vi "trialsExp.vi"() -> ()   [LabVIEW 2010]
uses:
  <instrlib>/niHWS/nihws.llb/niHWS Open File Permissions ID.ctl
  Statechart 1.lvsc/Trigger.ctl
  Statechart 1.lvsc/Inputs.ctl
  <vilib>/sound2/lvsound2.llb/Sound Data Format.ctl
  <vilib>/sound2/lvsound2.llb/Sampling Mode.ctl
  <vilib>/Statechart/Infrastructure/RTStatechart/RunTime SCN.xnode
  Statechart 1.lvsc/Outputs.ctl
  Statechart 1.lvsc
  <vilib>/Statechart/Common/IntGuid.ctl
  <vilib>/Statechart/Common/DbgID.ctl
  <vilib>/DAQmx/write.llb/DAQmx Write (Digital Bool 1Line 1Point).vi
  <instrlib>/niHWS/nihws.llb/niHWS Write Analog DBL.vi
  <vilib>/imath/engines/lvmath2/RunTimeEngine/ErrorHandling/NIMS_Finalize Error.vi
  <vilib>/imath/engines/lvmath2/RunTimeEngine/NodeEndStatement/NIMS_NodeEndStatement_Get Vector.vi
  <instcachedir>/0/NIMS_NodeEndStatement_Get Vector_F420F1081A35401FA339BC91980782B0.lvgen/NIMS_NodeEndStatement_Get Vector_F420F1081A35401FA339BC91980782B0_002.vi
  <vilib>/imath/engines/lvmath/Functions/Error Handling/MergeErrorsWrapper.vi
  <vilib>/imath/engines/lvmath2/RunTimeEngine/NodeEndStatement/NIMS_NodeEndStatement_Output.vi
  <instcachedir>/0/NIMS_NodeEndStatement_Output_53EC0D466D134D7ABD903AC30B43404B.lvgen/NIMS_NodeEndStatement_Output_53EC0D466D134D7ABD903AC30B43404B_004.vi
  <instcachedir>/0/NIMS_NodeEndStatement_Output_53EC0D466D134D7ABD903AC30B43404B.lvgen/NIMS_NodeEndStatement_Output_53EC0D466D134D7ABD903AC30B43404B_005.vi
  <vilib>/imath/engines/lvmath2/RunTimeEngine/RangeToken/NIMS_Range.vi
  <instcachedir>/0/NIMS_Range_1C63927E4E474DADACDA97C3F2261A11.lvgen/NIMS_Range_1C63927E4E474DADACDA97C3F2261A11_000.vi
  <vilib>/imathl/engines/lvmath/Functions/Error Handling/Create Error.vi
  <vilib>/imath/engines/lvmath2/RunTimeEngine/BuiltInFunctions/repeatmx/NIMS_repeatmx(GM, I32, I32).vi
  <instcachedir>/0/NIMS_repeatmx(GM, I32, I32)_69DEE8FEFC4F4D9AB51BA55E85245ECE.lvgen/NIMS_repeatmx(GM, I32, I32)_69DEE8FEFC4F4D9AB51BA55E85245ECE_004.vi
  <vilib>/imath/engines/lvmath2/RunTimeEngine/BuiltInFunctions/randpermutation/NIMS_randpermutation.vi
  <vilib>/imath/engines/lvmath2/RunTimeEngine/VariableToken/Read/NIMS_Get Elements - SorM(_) - Check.vi
  <instcachedir>/0/NIMS_Get Elements - SorM(_) - Check_404BE36992094B78AAADB7BD5278D7E3.lvgen/NIMS_Get Elements - SorM(_) - Check_404BE36992094B78AAADB7BD5278D7E3_006.vi
  <vilib>/sound2/lvsound2.llb/Sound Output Write (DBL Single).vi
  Statechart 1.lvsc/CompanionDiagram.vi/21/SC Main.vi
  <vilib>/daqmx/miscellaneous.llb/DAQmx Fill In Error Info.vi
  <vilib>/measure/NI_MABase.lvlib
  <vilib>/Statechart/Common/NI_SC_LVSCCommonFiles.lvlib
panel:
  in  "Tab Control":T1(tab)
  in  "Mouse Axis":bool
  in  "DPI":dbl=400.0
  in  "Mouse ID":refnum<visa-resource-name>
  in  "Recording Path":path
  out "Stimulus Parameters":string[](array[string])
  in  "Param Array":dbl[][](array[numeric])
  in  "Stimuli":string[](array[combo])
  in  "Performance\nAverage trials":dbl=10.0
  out "Total Trials":dbl
  out "Stim":dbl[](array[numeric])
  out "expInd":dbl[](array[numeric])
  out "CurrCond":dbl
  out "Terminate":bool
  out "Now Showing":string
  out "Number of Conditions":u32
  out "Trial Params":T2
  out "Writing \nto File":bool
  out "Audio\nPeriod":bool
  out "Wait Period":bool
  out "ActivitySum":dbl format="%#_3g"
  out "Audio":bool
  out "Juice":bool
  out "Elapsed Time (s)":dbl format="%#_2g"
  out "Iteration":dbl
  out "Shock":bool
  out "Activity":dynamicdata(graph) caption="Collected Signals"
  in  "stop":bool
  in  "START":bool
  out "Waveform Graph":dynamicdata(graph)
  out "corrects 1":dbl
  out "wrongs 1":dbl
  out "corrects 2":dbl
  out "wrongs 2":dbl
  in  "Params":T3(array[cluster])
  out "element":T2
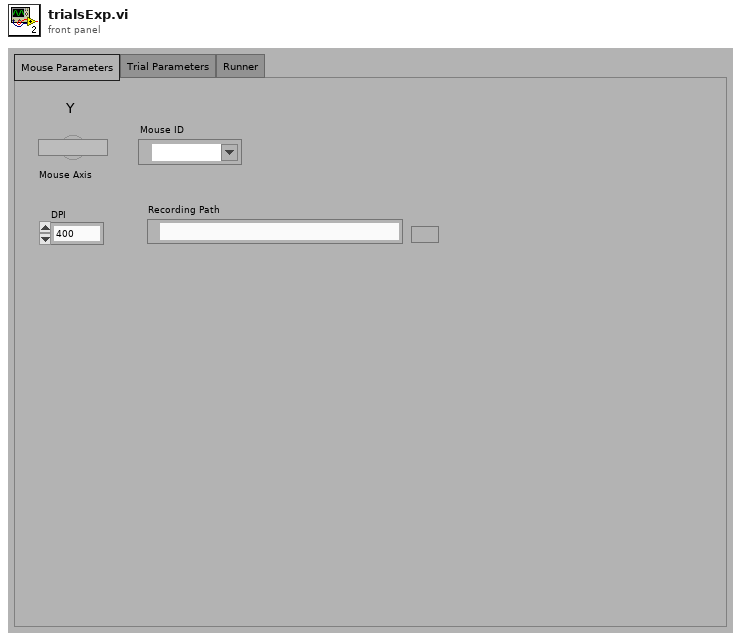
[diagram p1: front panel]
types:
  T1 = enum32{"Mouse Parameters", "Trial Parameters", "Runner"}
  T2 = cluster{"Frequency":dbl, "Pattern Freq":dbl, "ITI":dbl, "Audio Duration":dbl, "Audio Delay":dbl, "Shock Duration":dbl, "Repeat #":dbl, "Juice Duration":dbl, "Activity Thr":dbl}
  T3 = cluster{"Frequency":dbl, "Pattern Freq":dbl, "ITI":dbl, "Audio\n Duration":dbl, "Audio Delay":dbl, "Shock Duration":dbl, "Repeat #":dbl, "Juice Duration":dbl, "Activity Thr":dbl}[]
  T4 = typedef "niHWS Open File Permissions ID.ctl" = enum32{"Read Only", "Read/Write Existing", "Read/Write/Create New", "Read/Write/Create New Always"}
  T5 = cluster{"Frequency":dbl, "Pattern Freq":dbl, "ITI":dbl, "Audio Duration":dbl, "Audio Delay":dbl, "Shock Duration":dbl, "Repeat #":dbl, "Juice Duration":dbl, "Activity Thr":dbl}[]
  T6 = typedef "Statechart 1.lvsc/Inputs.ctl" = cluster{"Audio Duration":dbl, "Shock Duration ":dbl, "Audio Delay":dbl, "timer":dbl, "Iteration":dbl, "clearTime":dbl, "ITI":dbl, "MaxTrials":dbl, "Juice Duration":dbl, "Activity":dbl, "Activity Thr":dbl}
  T7 = typedef "NI_SC_LVSCCommonFiles.lvlib/IntGuid.ctl" = cluster{"Data1":u32, "Data2":u16, "Data3":u16, "Data4":u8, "Data5":u8, "Data6":u8, "Data11":u8, "Data9":u8, "Data10":u8, "Data8":u8, "Data7":u8}
  T8 = typedef "NI_SC_LVSCCommonFiles.lvlib/DbgID.ctl" = cluster{"VIRef":u32, "IntGUID":T7}
  T9 = cluster{"Frequency":dbl, "Pattern Freq":dbl, "ITI":dbl, "Audio\n Duration":dbl, "Audio Delay":dbl, "Shock Duration":dbl, "Repeat #":dbl, "Juice Duration":dbl, "Activity Thr":dbl}
  T10 = typedef "Sound Data Format.ctl" = cluster{"sample rate (S/s)":dbl, "number of channels":i32, "bits per sample":i32}
  T11 = typedef "Sampling Mode.ctl" = i32
  T12 = typedef "Sound Output Task ID.ctl" = u32
  T13 = typedef "Statechart 1.lvsc/Outputs.ctl" = cluster{"Iteration":dbl, "Audio":bool, "Shock":bool, "clearTime":dbl, "Juice":bool, "correct":dbl, "Wait Period":bool}
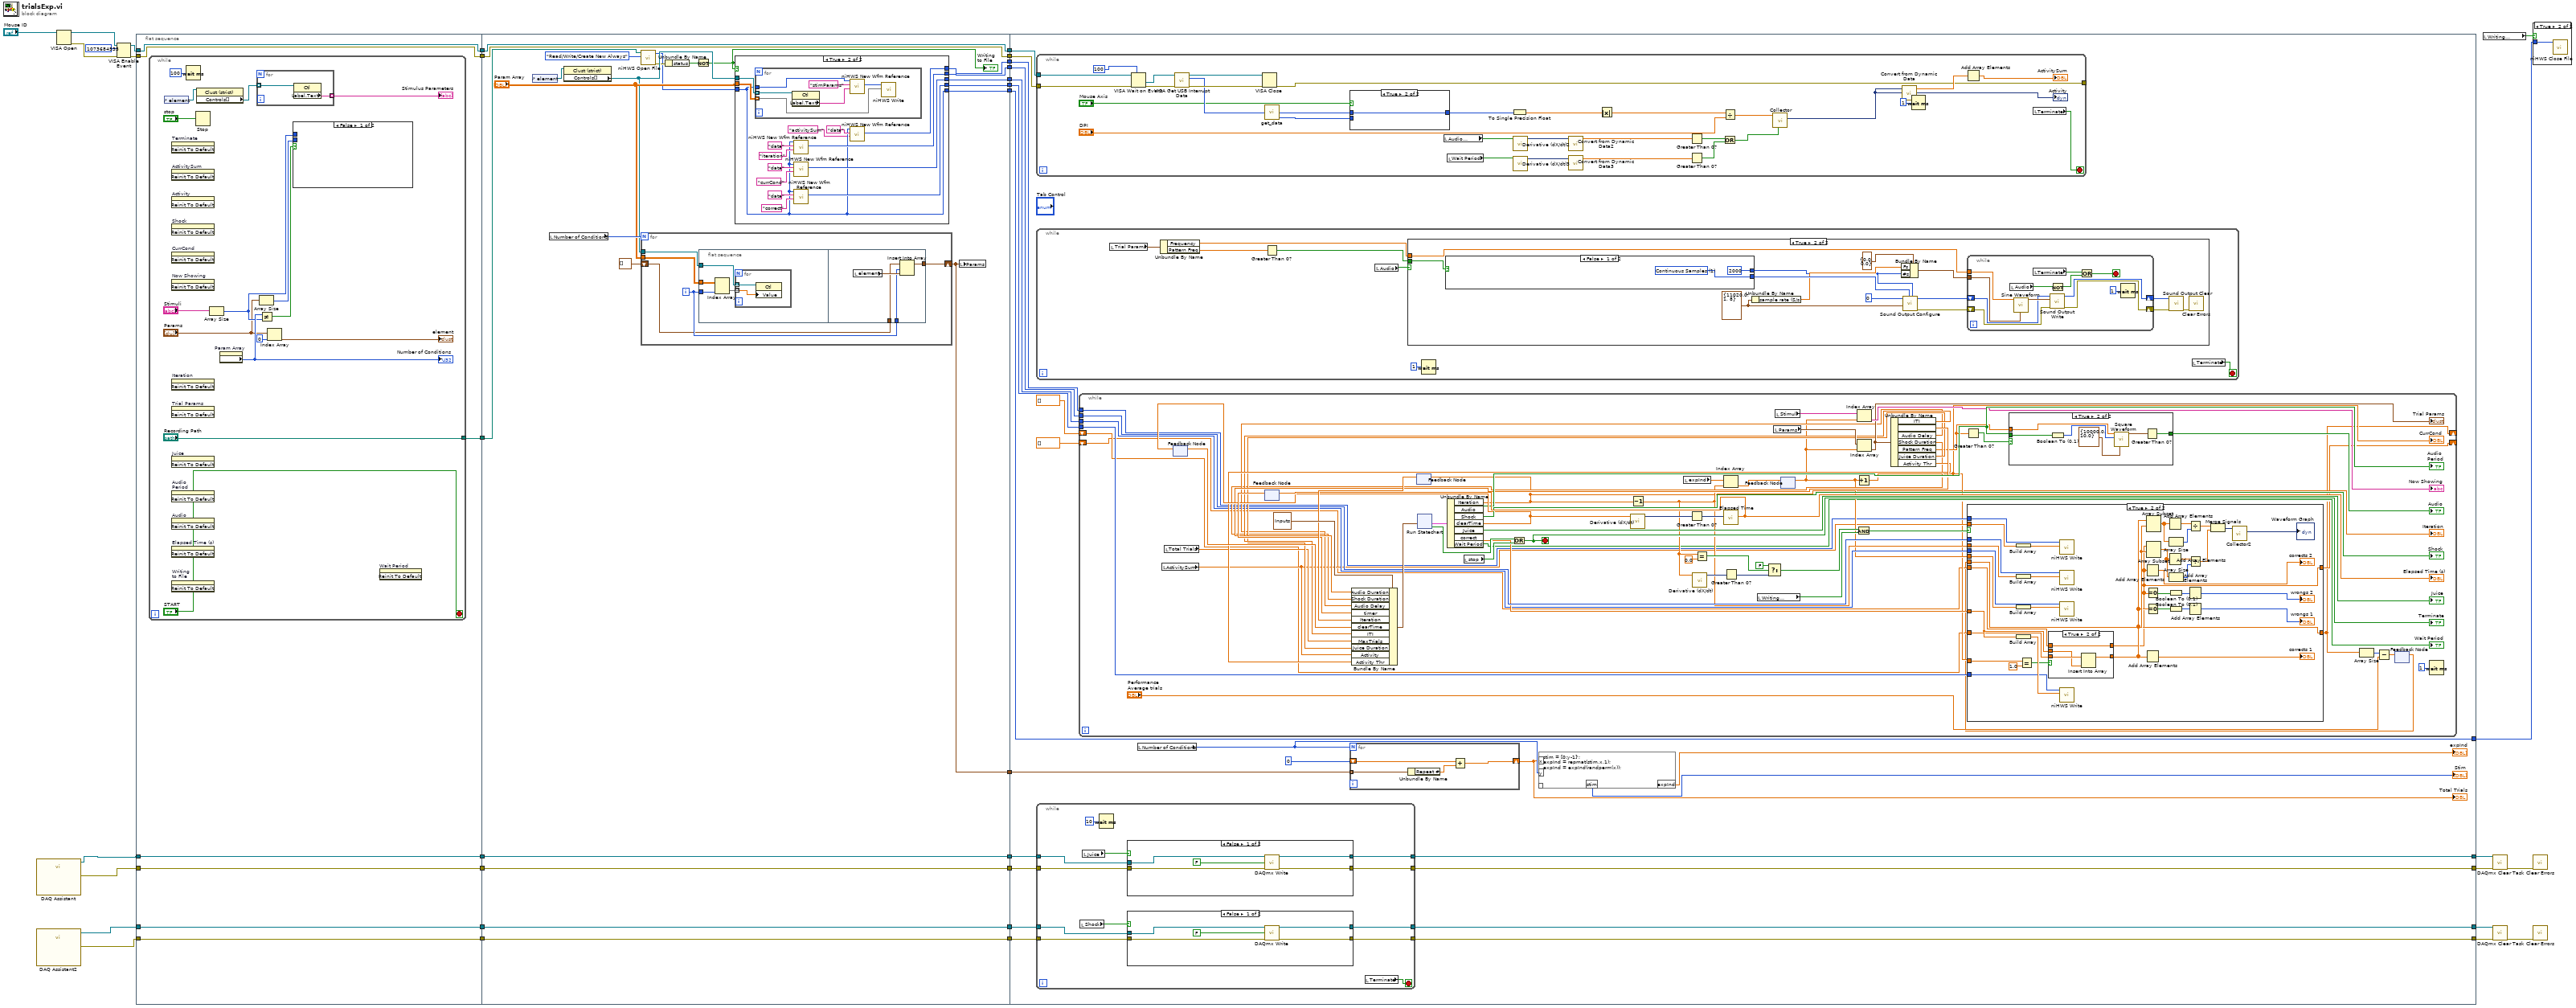
[diagram p0: block diagram]
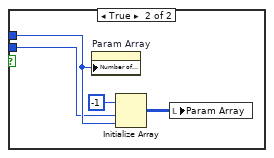
[diagram p3: hidden frame]
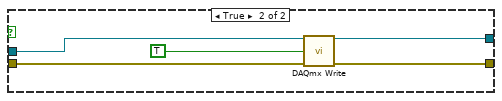
[diagram p6: hidden frame]
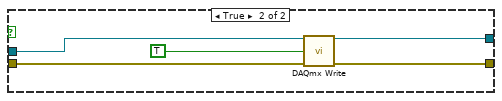
[diagram p7: hidden frame]
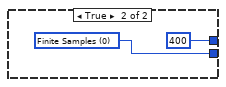
[diagram p9: hidden frame]
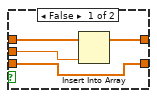
[diagram p11: hidden frame]
diagram:
  n1 = call "DAQ Assistant"() -> ("task out"=w4:refnum<k21>, "error out"=w3:errorcluster)  [unwired: 18 in]
  n2 = call "DAQ Assistant2"() -> ("task out"=w2:refnum<k21>, "error out"=w1:errorcluster)  [unwired: 18 in]
  n3 = VISA Open(VISA resource name="Mouse ID") -> (VISA resource name=w20:refnum<visa-resource-name>, error out=w21:errorcluster)  [unwired: 1 in, 3 out]
  n4 = VISA Enable Event(8:w21, 10:u32 1073684535 ("event type"), 11:w20) -> (0:w18:errorcluster, 3:w19:refnum<visa-resource-name>)  [unwired: 1 out]
  n5 = flat-sequence {
    tunnel: [w44] -> w37
    tunnel: w2 -> [w44]
    tunnel: [w43] -> w36
    tunnel: w4 -> [w43]
    tunnel: [w42] -> w35
    tunnel: w19 -> [w42]
    tunnel: [w41] -> w34
    tunnel: w18 -> [w41]
    tunnel: [w40] -> w33
    tunnel: w1 -> [w40]
    tunnel: [w39] -> w32
    tunnel: w3 -> [w39]
    tunnel: [w38] -> w12
    tunnel: w37 -> [w88]
    tunnel: [w88] -> w31
    tunnel: w36 -> [w87]
    tunnel: [w87] -> w30
    tunnel: w35 -> [w86]
    tunnel: [w86] -> w29
    tunnel: w34 -> [w85]
    tunnel: [w85] -> w28
    tunnel: w33 -> [w84]
    tunnel: [w84] -> w27
    tunnel: w32 -> [w83]
    tunnel: [w83] -> w26
    tunnel: [w82] -> w25
    tunnel: w12 -> [w76]
    tunnel: [w70] -> w11
    tunnel: [w69] -> w10
    tunnel: [w68] -> w9
    tunnel: [w67] -> w8
    tunnel: [w66] -> w5
    tunnel: w31 -> [w146]
    tunnel: w30 -> [w139]
    tunnel: [w145] -> w24
    tunnel: [w137] -> w23
    tunnel: w29 -> [w144]
    tunnel: w28 -> [w143]
    tunnel: w27 -> [w142]
    tunnel: w26 -> [w138]
    tunnel: [w141] -> w17
    tunnel: [w136] -> w16
    tunnel: w25 -> [w134]
    tunnel: w11 -> [w131]
    tunnel: w10 -> [w130]
    tunnel: w9 -> [w128]
    tunnel: w8 -> [w129]
    tunnel: [w128] -> w7
    tunnel: w5 -> [w127]
    frame #0 {
      n6 = while {
        tunnel: ["Recording Path"] -> w38
        stop <- "START" stop-if-true
        n7 = control-ref of="element"() -> (w53:refnum<vi>)
        n8 = invoke on="Terminate" class="Bool (strict)" method="Reinit To Default"() -> ()  [unwired: 3 in, 3 out]
        n9 = invoke on="ActivitySum" class="DigNum (strict)" method="Reinit To Default"() -> ()  [unwired: 3 in, 3 out]
        n10 = invoke on="Activity" class="WFGraph (strict)" method="Reinit To Default"() -> ()  [unwired: 3 in, 3 out]
        n11 = invoke on="Shock" class="Bool (strict)" method="Reinit To Default"() -> ()  [unwired: 3 in, 3 out]
        n12 = invoke on="CurrCond" class="DigNum (strict)" method="Reinit To Default"() -> ()  [unwired: 3 in, 3 out]
        n13 = invoke on="Now Showing" class="Str" method="Reinit To Default"() -> ()  [unwired: 3 in, 3 out]
        n14 = invoke on="Iteration" class="DigNum (strict)" method="Reinit To Default"() -> ()  [unwired: 3 in, 3 out]
        n15 = invoke on="Trial Params" class="Clust (strict)" method="Reinit To Default"() -> ()  [unwired: 3 in, 3 out]
        n16 = invoke on="Juice" class="Bool (strict)" method="Reinit To Default"() -> ()  [unwired: 3 in, 3 out]
        n17 = invoke on="Audio\nPeriod" class="Bool (strict)" method="Reinit To Default"() -> ()  [unwired: 3 in, 3 out]
        n18 = invoke on="Audio" class="Bool (strict)" method="Reinit To Default"() -> ()  [unwired: 3 in, 3 out]
        n19 = invoke on="Elapsed Time (s)" class="DigNum (strict)" method="Reinit To Default"() -> ()  [unwired: 3 in, 3 out]
        n20 = invoke on="Writing \nto File" class="Bool (strict)" method="Reinit To Default"() -> ()  [unwired: 3 in, 3 out]
        n21 = Wait (ms)(milliseconds to wait=100) -> ()  [unwired: 1 out]
        n22 = Stop(stop? (T)="stop") -> ()
        n23 = property class="Clust (strict)"(reference=w53) -> ("Controls[]"=w52:refnum<vi>[])  [unwired: 1 in, 2 out]
        n24 = Array Size(array="Stimuli") -> (size(s)=w50:i32)
        n25 = property on="Param Array" class="Arr (strict)"() -> ("Number of Columns"=w59:u32)  [unwired: 2 in, 2 out]
        "Number of Conditions" <- w59
        n26 = for {
          tunnel: w52 -> [w61] mode=indexing
          tunnel: [w60] -> w51 mode=indexing
          n27 = property class="Ctl"(reference=w61) -> ("Label.Text"=w60:string)  [unwired: 1 in, 2 out]
        }
        "Stimulus Parameters" <- w51
        n28 = Array Size(array="Params") -> (size(s)=w54:i32)
        n29 = Not Equal?(x=w59, y=w50) -> (x != y?=w58:bool)
        n30 = Index Array(array="Params", index=0) -> (element=→"element":T9)
        n31 = case shown="False" w58 {
          tunnel: w50 -> [_ w63]
          tunnel: w54 -> [_ w62]
          frame False {
          }
          frame True {
            n32 = property on="Param Array" class="Arr (strict)"("Number of Columns"=w63) -> ()  [unwired: 2 in, 2 out]
            n33 = Initialize Array(-1, w62, w63) -> (w64:i32[][])
            n34 = local write "Param Array"(w64) -> ()
          }
        }
        n35 = invoke on="Wait Period" class="Bool (strict)" method="Reinit To Default"() -> ()  [unwired: 3 in, 3 out]
      }
    }
    frame #1 {
      n36 = control-ref of="element"() -> (w78:refnum<vi>)
      n37 = local read "Number of Conditions"() -> (w80:u32)
      n38 = property class="Clust (strict)"(reference=w78) -> ("Controls[]"=w77:refnum<vi>[])  [unwired: 1 in, 2 out]
      n39 = call <instrlib>:"niHWS Open File.vi"("permissions (0:read only)"=niHWS_Open_File_Permissions_ID."Read/Write/Create New Always", "file path"=w76) -> ("error out"=w74:errorcluster, "file handle"=w71:u32)  [unwired: 8 in]
      n40 = for {
        N: w80 -> [_]
        tunnel: "Param Array" -> [w113]
        shift-right: [w111] -> w82
        shift-left: T5 [] ("array") -> [w112]
        tunnel: w77 -> [w110]
        i -> [w114]
        n41 = flat-sequence {
          tunnel: w113 -> [w116]
          tunnel: w114 -> [w117]
          tunnel: w110 -> [w115]
          tunnel: w112 -> [w122]
          tunnel: w114 -> [w123]
          tunnel: [w121] -> w111
          frame #0 {
            n42 = Index Array(array=w116, index (col)=w117) -> (element=w118:dbl[])  [unwired: 1 in]
            n43 = for {
              tunnel: w115 -> [w119] mode=indexing
              tunnel: w118 -> [w120] mode=indexing
              n44 = property class="Ctl"(reference=w119, "Value"=w120) -> ()  [unwired: 1 in, 2 out]
            }
          }
          frame #1 {
            n45 = local read "element"() -> (w124:T2)
            n46 = Insert Into Array(array=w122, index=w123, new element=w124) -> (w121:T5)
          }
        }
      }
      n47 = Unbundle By Name(w74) -> ("status"=w73:bool)
      n48 = Not(x=w73) -> (.not. x?=w72:bool)
      "Writing \nto File" <- w72
      n49 = case shown="True" w72 {
        tunnel: "Param Array" -> [_ w103]
        tunnel: w77 -> [_ w102]
        tunnel: w71 -> [_ w91]
        tunnel: [_ w95] -> w70
        tunnel: [_ w94] -> w69
        tunnel: [_ w93] -> w67
        tunnel: [_ w91] -> w68
        tunnel: [_ w89] -> w66
        frame False {
        }
        frame True {
          n50 = for {
            tunnel: w102 -> [w109] mode=indexing
            tunnel: w103 -> [w105] mode=indexing
            tunnel: w91 -> [w104]
            n51 = property class="Ctl"(reference=w109) -> ("Label.Text"=w108:string)  [unwired: 1 in, 2 out]
            n52 = call <instrlib>:"niHWS New Wfm Reference.vi"("waveform name (empty)"=w108, "group name (empty)"="stimParams", "file handle in"=w104) -> ("waveform reference"=w106:u32)  [unwired: 6 in, 2 out]
            n53 = call-poly <instrlib>:"niHWS Write.vi"("data"=w105, "waveform reference in"=w106) -> ()  [unwired: 8 in, 2 out]
          }
          n54 = call <instrlib>:"niHWS New Wfm Reference.vi"("waveform name (empty)"="iteration", "group name (empty)"="data", "file handle in"=w91) -> ("waveform reference"=w95:u32)  [unwired: 6 in, 2 out]
          n55 = call <instrlib>:"niHWS New Wfm Reference.vi"("waveform name (empty)"="currCond", "group name (empty)"="data", "file handle in"=w91) -> ("waveform reference"=w94:u32)  [unwired: 6 in, 2 out]
          n56 = call <instrlib>:"niHWS New Wfm Reference.vi"("waveform name (empty)"="correct", "group name (empty)"="data", "file handle in"=w91) -> ("waveform reference"=w93:u32)  [unwired: 6 in, 2 out]
          n57 = call <instrlib>:"niHWS New Wfm Reference.vi"("waveform name (empty)"="activitySum", "group name (empty)"="data", "file handle in"=w91) -> ("waveform reference"=w89:u32)  [unwired: 6 in, 2 out]
        }
      }
      n58 = local write "Params"(w82) -> ()
    }
    frame #2 {
      n59 = while {
        tunnel: w144 -> [w182]
        tunnel: w143 -> [w181]
        tunnel: [w160] -> _
        stop <- w177 stop-if-true
        n60 = VISA Wait on Event(7:u32 100 ("timeout (0)"), 8:w181, 11:w182) -> (0:w178:errorcluster, 1:w179:refnum<visa-resource-name>)  [unwired: 4 out]
        n61 = call <vilib>:"VISA Get USB Interrupt Data.vi"("error in (no error)"=w178, "VISA USB Intr Event"=w179) -> ("error out"=w174:errorcluster, "data buffer"=w173:u8[], "VISA USB Intr Event out"=w175:refnum<visa-resource-name>)  [unwired: 7 out]
        n62 = VISA Close(VISA resource name=w175, error in (no error)=w174) -> (error out=w160:errorcluster)
        n63 = call "get_data.vi"("data buffer"=w173) -> ("X Value"=w171:i8, "Y Value"=w170:i8)  [unwired: 1 out]
        n64 = case shown="True" "Mouse Axis" {
          tunnel: w171 -> [_ w184]
          tunnel: [w183 w184] -> w167
          tunnel: w170 -> [w183 _]
          frame False {
          }
          frame True {
          }
        }
        n65 = local read "Audio\nPeriod"() -> (w161:bool)
        n66 = local read "Wait Period"() -> (w155:bool)
        n67 = To Single Precision Float(number=w167) -> (single precision float=w163:sgl)
        n68 = call "Derivative (dX/dt)2"("Signals"=w161) -> ("Result"=w159:dynamicdata)  [unwired: 5 in, 1 out]
        n69 = call "Derivative (dX/dt)3"("Signals"=w155) -> ("Result"=w154:dynamicdata)  [unwired: 5 in, 1 out]
        n70 = call "Convert from Dynamic Data2"("Dynamic Data Type"=w159) -> ("Scalar"=w158:dbl)  [unwired: 3 in]
        n71 = call "Convert from Dynamic Data3"("Dynamic Data Type"=w154) -> ("Scalar"=w153:dbl)  [unwired: 3 in]
        n72 = Absolute Value(x=w163) -> (abs(x)=w162:sgl)
        n73 = Greater Than 0?(x=w158) -> (x > 0?=w157:bool)
        n74 = Greater Than 0?(x=w153) -> (x > 0?=w152:bool)
        n75 = Or(x=w157, y=w152) -> (x .or. y?=w156:bool)
        n76 = Divide(x=w162, y="DPI") -> (x/y=w168:dbl)
        n77 = call "Collector"("Reset"=w156, "Signals"=w168) -> ("Collected Signals"=w166:dynamicdata)  [unwired: 8 in, 1 out]
        "Activity" <- w166
        n78 = call "Convert from Dynamic Data"("Dynamic Data Type"=w166) -> ("Array"=w165:dbl[])  [unwired: 3 in]
        n79 = Wait (ms)(milliseconds to wait=1) -> ()  [unwired: 1 out]
        n80 = Add Array Elements(numeric array=w165) -> (sum=→"ActivitySum":dbl)
        n81 = local read "Terminate"() -> (w177:bool)
      }
      n82 = while {
        stop <- w223 stop-if-true
        n83 = local read "Trial Params"() -> (w219:T2)
        n84 = Unbundle By Name(w219) -> ("Frequency"=w218:dbl, "Pattern Freq"=w217:dbl)
        n85 = Greater Than 0?(x=w217) -> (x > 0?=w220:bool)
        n86 = local read "Audio"() -> (w222:bool)
        n87 = case shown="True" w222 {
          tunnel: w218 -> [_ w227]
          tunnel: w220 -> [_ w225]
          frame False {
          }
          frame True {
            w230 = T10 {"sample rate (S/s)"=11020.0, "number of channels"=1, "bits per sample"=8} ("Sound Format")
            n88 = case shown="False" w225 {
              tunnel: [w239 w241] -> w234
              tunnel: [2000 ("Number of Samples/ch") 400 ("Number of Samples/ch")] -> w224
              frame False {
                w239 = T11 1 items=["Finite Samples", "Continuous Samples"] ("sample mode")
              }
              frame True {
                w241 = T11 0 items=["Finite Samples", "Continuous Samples"] ("sample mode")
              }
            }
            n89 = Unbundle By Name(w230) -> ("sample rate (S/s)"=w231:dbl)
            n90 = Bundle By Name(cluster=cluster{"Fs":dbl, "#s":dbl} {"Fs"=0.0, "#s"=0.0} ("sampling info"), "Fs"=w231, "#s"=w224) -> (w232:cluster{"Fs":dbl, "#s":dbl})
            n91 = call <vilib>:"Sound Output Configure.vi"("number of samples/ch"=w224, "sample mode"=w234, "sound format"=w230, "device ID"=u32 0 ("Device ID")) -> ("error out"=w237:errorcluster, "task ID"=w236:T12)  [unwired: 6 in]
            n92 = while {
              shift-right: [w252] -> w228
              shift-left: w237 -> [w248]
              shift-right: [w253] -> w229
              shift-left: w236 -> [w249]
              tunnel: w232 -> [w251]
              tunnel: w227 -> [w247]
              stop <- w246 stop-if-true
              n93 = local read "Audio"() -> (w243:bool)
              n94 = call <vilib>:"Sine Waveform.vi"("sampling info"=w251, "frequency"=w247) -> ("signal out"=w250:waveform(dbl))  [unwired: 8 in, 1 out]
              n95 = local read "Terminate"() -> (w244:bool)
              n96 = call-poly <vilib>:"Sound Output Write.vi"("error in (no error)"=w248, "data"=w250, "task ID"=w249) -> ("error out"=w252:errorcluster, "task ID out"=w253:T12)  [unwired: 7 in]
              n97 = Not(x=w243) -> (.not. x?=w245:bool)
              n98 = Or(x=w244, y=w245) -> (x .or. y?=w246:bool)
              n99 = Wait (ms)(milliseconds to wait=1) -> ()  [unwired: 1 out]
            }
            n100 = call <vilib>:"Sound Output Clear.vi"("error in (no error)"=w228, "task ID"=w229) -> ("error out"=w226:errorcluster)  [unwired: 9 in]
            n101 = call <vilib>:"Clear Errors.vi"("error in (no error)"=w226) -> ()  [unwired: 6 in, 1 out]
          }
        }
        n102 = Wait (ms)(milliseconds to wait=1) -> ()  [unwired: 1 out]
        n103 = local read "Terminate"() -> (w223:bool)
      }
      n104 = while {
        tunnel: w146 -> [w196]
        tunnel: [w195] -> w145
        tunnel: w142 -> [w192]
        tunnel: [w191] -> w141
        tunnel: w139 -> [w189]
        tunnel: w138 -> [w188]
        tunnel: [w187] -> w137
        tunnel: [w186] -> w136
        stop <- w193 stop-if-true
        n105 = local read "Shock"() -> (w194:bool)
        n106 = local read "Juice"() -> (w190:bool)
        n107 = Wait (ms)(milliseconds to wait=10) -> ()  [unwired: 1 out]
        n108 = case shown="False" w190 {
          tunnel: w189 -> [w200 w206]
          tunnel: [w199 w204] -> w187
          tunnel: w188 -> [w198 w203]
          tunnel: [w197 w202] -> w186
          frame False {
            n109 = call-poly <vilib>:"DAQmx Write.vi"("task/channels in"=w200, "data"=FALSE, "error in"=w198) -> ("task out"=w199:refnum<k21>, "error out"=w197:errorcluster)  [unwired: 10 in, 1 out]
          }
          frame True {
            n110 = call-poly <vilib>:"DAQmx Write.vi"("task/channels in"=w206, "data"=TRUE, "error in"=w203) -> ("task out"=w204:refnum<k21>, "error out"=w202:errorcluster)  [unwired: 10 in, 1 out]
          }
        }
        n111 = case shown="False" w194 {
          tunnel: w196 -> [w210 w216]
          tunnel: [w209 w214] -> w195
          tunnel: w192 -> [w208 w213]
          tunnel: [w207 w212] -> w191
          frame False {
            n112 = call-poly <vilib>:"DAQmx Write.vi"("task/channels in"=w210, "data"=FALSE, "error in"=w208) -> ("task out"=w209:refnum<k21>, "error out"=w207:errorcluster)  [unwired: 10 in, 1 out]
          }
          frame True {
            n113 = call-poly <vilib>:"DAQmx Write.vi"("task/channels in"=w216, "data"=TRUE, "error in"=w213) -> ("task out"=w214:refnum<k21>, "error out"=w212:errorcluster)  [unwired: 10 in, 1 out]
          }
        }
        n114 = local read "Terminate"() -> (w193:bool)
      }
      n115 = while {
        tunnel: w131 -> [w277]
        tunnel: w130 -> [w275]
        tunnel: w129 -> [w274]
        tunnel: w127 -> [w264]
        shift-right: [w257] -> _
        shift-left: dbl[] [] ("array") -> [w262]
        shift-right: [w258] -> _
        shift-left: dbl[] [] ("array") -> [w261]
        stop <- w302 stop-if-true
        n116 = local read "ActivitySum"() -> (w265:dbl)
        n117 = local read "Total Trials"() -> (w283:dbl)
        n118 = feedback #1() -> (w304:dbl)  [unwired: 1 in]
        n119 = feedback #2() -> (w310:dbl)  [unwired: 1 in]
        n120 = feedback #3() -> (w312:dbl)  [unwired: 1 in]
        n121 = local read "stop"() -> (w294:bool)
        n122 = local read "expInd"() -> (w282:dbl[])
        n123 = local read "Writing \nto File"() -> (w279:bool)
        n124 = local read "Params"() -> (w295:T3)
        n125 = local read "Stimuli"() -> (w293:string[])
        n126 = feedback #4() -> (w267:dbl)  [unwired: 1 in]
        n127 = Increment(x=w267) -> (x+1=w263:dbl)
        "CurrCond" <- w263
        n128 = Index Array(array=w293, index=w267) -> (element=→"Now Showing":string)
        n129 = Index Array(array=w295, index=w267) -> (element=w291:T9)
        "Trial Params" <- w291
        n130 = Unbundle By Name(w291) -> ("ITI"=w288:dbl, "Audio\n Duration"=w290:dbl, "Audio Delay"=w286:dbl, "Shock Duration"=w285:dbl, "Pattern Freq"=w284:dbl, "Juice Duration"=w287:dbl, "Activity Thr"=w289:dbl)
        n131 = Bundle By Name(cluster=T6 {"Audio Duration"=0.0, "Shock Duration "=0.0, "Audio Delay"=0.0, "timer"=0.0, "Iteration"=0.0, "clearTime"=0.0, "ITI"=0.0, "MaxTrials"=0.0, "Juice Duration"=0.0, "Activity"=0.0, "Activity Thr"=0.0} ("Inputs"), "Audio Duration"=w290, "Shock Duration"=w285, "Audio Delay"=w286, "timer"=w310, "Iteration"=w312, "clearTime"=w304, "ITI"=w288, "MaxTrials"=w283, "Juice Duration"=w287, "Activity"=w265, "Activity Thr"=w289) -> (w306:T6)
        n132 = xnode "Run Statechart"("Inputs"=w306) -> ("Terminated?"=w301:bool, "Outputs"=w305:T13)  [unwired: 2 in]
        n133 = Unbundle By Name(w305) -> ("Iteration"=w260:dbl, "Audio"=w299:bool, "Shock"=→"Shock":bool, "clearTime"=w303:dbl, "Juice"=→"Juice":bool, "correct"=w276:dbl, "Wait Period"=→"Wait Period":bool)
        "Iteration" <- w260
        "Audio\nPeriod" <- w299
        n134 = feedback-in #1(w303) -> ()
        n135 = feedback-in #3(w260) -> ()
        n136 = Or(x=w301, y=w294) -> (x .or. y?=w302:bool)
        "Terminate" <- w302
        n137 = call "Derivative (dX/dt)"("Signals"=w303) -> ("Result"=w309:dynamicdata)  [unwired: 5 in, 1 out]
        n138 = Decrement(x=w260) -> (x-1=w268:dbl)
        n139 = Greater Than 0?(x=w309) -> (x > 0?=w308:dynamicdata)
        n140 = call "Derivative (dX/dt)"("Signals"=w268) -> ("Result"=w280:dynamicdata)  [unwired: 5 in, 1 out]
        n141 = Equal?(x=w268, y=0.0) -> (x = y?=w270:bool)
        n142 = Index Array(array=w282, index=w268) -> (element=w281:dbl)
        n143 = call "Elapsed Time"("Reset"=w308) -> ("Elapsed Time (s)"=w311:dbl)  [unwired: 11 in, 7 out]
        "Elapsed Time (s)" <- w311
        n144 = feedback-in #2(w311) -> ()
        n145 = Greater Than 0?(x=w280) -> (x > 0?=w273:dynamicdata)
        n146 = Select(t=FALSE, s=w270, f=w273) -> (s? t:f=w272:bool)
        n147 = feedback-in #4(w281) -> ()
        n148 = And(x=w272, y=w279) -> (x .and. y?=w278:bool)
        n149 = Greater Than 0?(x=w284) -> (x > 0?=w296:bool)
        n150 = case shown="True" w296 {
          tunnel: w299 -> [w362 w368]
          tunnel: w284 -> [_ w366]
          tunnel: [w362 w363] -> w297
          frame False {
          }
          frame True {
            n151 = Boolean To (0,1)(Boolean=w368) -> (0, 1=w367:i16)
            n152 = call <vilib>:"Square Waveform.vi"("sampling info"=cluster{"Fs":dbl, "#s":dbl} {"Fs"=10000.0, "#s"=10.0}, "amplitude"=w367, "frequency"=w366) -> ("signal out"=w364:waveform(dbl))  [unwired: 7 in, 1 out]
            n153 = Greater Than 0?(x=w364) -> (x > 0?=w363:bool)
          }
        }
        "Audio" <- w297
        n154 = feedback #5() -> (w254:dbl)  [unwired: 1 in]
        n155 = case shown="True" w278 {
          tunnel: w268 -> [_ w352]
          tunnel: w277 -> [_ w353]
          tunnel: w267 -> [_ w348]
          tunnel: w276 -> [_ w339]
          tunnel: w275 -> [_ w347]
          tunnel: w274 -> [_ w346]
          tunnel: w265 -> [_ w344]
          tunnel: w264 -> [_ w343]
          tunnel: w263 -> [_ w341]
          tunnel: w262 -> [w315 w338]
          tunnel: w261 -> [w314 w337]
          tunnel: [w315 w324] -> w257
          tunnel: [w314 w318] -> w258
          tunnel: w254 -> [_ w330]
          frame False {
          }
          frame True {
            n156 = Build Array(w344) -> (w345:dbl[])
            n157 = Build Array(w352) -> (w351:dbl[])
            n158 = Build Array(w348) -> (w350:dbl[])
            n159 = Build Array(w339) -> (w349:dbl[])
            n160 = Equal?(x=w341, y=1.0) -> (x = y?=w340:bool)
            n161 = case shown="True" w340 {
              tunnel: w339 -> [w355 w359]
              tunnel: [w357 w361] -> w324
              tunnel: w338 -> [w357 w360]
              tunnel: w337 -> [w356 w358]
              tunnel: [w354 w358] -> w318
              frame False {
                n162 = Insert Into Array(array=w356, new element=w355) -> (w354:dbl[])  [unwired: 1 in]
              }
              frame True {
                n163 = Insert Into Array(array=w360, new element=w359) -> (w361:dbl[])  [unwired: 1 in]
              }
            }
            n164 = call-poly <instrlib>:"niHWS Write.vi"("data"=w345, "waveform reference in"=w343) -> ()  [unwired: 8 in, 2 out]
            n165 = call-poly <instrlib>:"niHWS Write.vi"("data"=w351, "waveform reference in"=w353) -> ()  [unwired: 8 in, 2 out]
            n166 = call-poly <instrlib>:"niHWS Write.vi"("data"=w350, "waveform reference in"=w347) -> ()  [unwired: 8 in, 2 out]
            n167 = call-poly <instrlib>:"niHWS Write.vi"("data"=w349, "waveform reference in"=w346) -> ()  [unwired: 8 in, 2 out]
            n168 = Add Array Elements(numeric array=w318) -> (sum=→"corrects 2":dbl)
            n169 = Add Array Elements(numeric array=w324) -> (sum=→"corrects 1":dbl)
            n170 = Equal To 0?(x=w318) -> (x = 0?=w320:bool[])
            n171 = Equal To 0?(x=w324) -> (x = 0?=w323:bool[])
            n172 = Array Subset(array=w324, index=w330) -> (w334:dbl[])  [unwired: 1 in]
            n173 = Array Subset(array=w318, index=w330) -> (w333:dbl[])  [unwired: 1 in]
            n174 = Add Array Elements(numeric array=w334) -> (sum=w335:dbl)
            n175 = Add Array Elements(numeric array=w333) -> (sum=w332:dbl)
            n176 = Boolean To (0,1)(Boolean=w320) -> (0, 1=w321:i16[])
            n177 = Boolean To (0,1)(Boolean=w323) -> (0, 1=w322:i16[])
            n178 = Array Size(array=w334) -> (size(s)=w336:i32)
            n179 = Array Size(array=w333) -> (size(s)=w331:i32)
            n180 = Divide(x=w335, y=w336) -> (x/y=w329:dbl)
            n181 = Divide(x=w332, y=w331) -> (x/y=w328:dbl)
            n182 = Add Array Elements(numeric array=w321) -> (sum=→"wrongs 2":i16)
            n183 = Add Array Elements(numeric array=w322) -> (sum=→"wrongs 1":i16)
            n184 = Merge Signals(w329, w328) -> (w327:dynamicdata)
            n185 = call "Collector2"("Signals"=w327) -> ("Collected Signals"=→"Waveform Graph":dynamicdata)  [unwired: 9 in, 1 out]
          }
        }
        n186 = Array Size(array=w257) -> (size(s)=w256:i32)
        n187 = Subtract(x=w256, y="Performance\nAverage trials") -> (x-y=w255:dbl)
        n188 = feedback-in #5(w255) -> ()
        n189 = Wait (ms)(milliseconds to wait=1) -> ()  [unwired: 1 out]
      }
      n190 = local read "Number of Conditions"() -> (w135:u32)
      n191 = for {
        N: w135 -> [_]
        tunnel: w134 -> [w151] mode=indexing
        shift-right: [w148] -> w132
        shift-left: 0 -> [w149]
        n192 = Unbundle By Name(w151) -> ("Repeat #"=w150:dbl)
        n193 = Add(x=w149, y=w150) -> (x+y=w148:dbl)
      }
      "Total Trials" <- w132
      n194 = mathscript code="stim = [0:y-1]';\nexpInd = repmat(stim,x,1);\nexpInd = expInd(randperm(x));"("x"=w132, "y"=w135) -> ("expInd"=→"expInd":dbl[], "stim"=→"Stim":i32[])  [unwired: 1 in, 1 out]
    }
  }
  n195 = local read "Writing \nto File"() -> (w6:bool)
  n196 = call <vilib>:"DAQmx Clear Task.vi"("task in"=w23, "error in"=w16) -> ("error out"=w14:errorcluster)  [unwired: 13 in]
  n197 = call <vilib>:"DAQmx Clear Task.vi"("task in"=w24, "error in"=w17) -> ("error out"=w15:errorcluster)  [unwired: 13 in]
  n198 = case shown="True" w6 {
    tunnel: w7 -> [_ w449]
    frame False {
    }
    frame True {
      n199 = call <instrlib>:"niHWS Close File.vi"("file handle"=w449) -> ()  [unwired: 10 in, 1 out]
    }
  }
  n200 = call <vilib>:"Clear Errors.vi"("error in (no error)"=w14) -> ()  [unwired: 6 in, 1 out]
  n201 = call <vilib>:"Clear Errors.vi"("error in (no error)"=w15) -> ()  [unwired: 6 in, 1 out]
